vi "Read Message Box.vi"(9 "MessageBox in":refnum<class "MessageBox.lvclass">) -> (3 "MessageBox out":refnum<class "MessageBox.lvclass">, 4 "Message Box":refnum<vi>)   [LabVIEW 2014, in "Raspberry Pi Compatible Compiler for LabVIEW.lvlib" / "MessageBox.lvclass"]
uses:
  MessageBox.lvclass
  MessageBox.lvclass/MessageBox.ctl
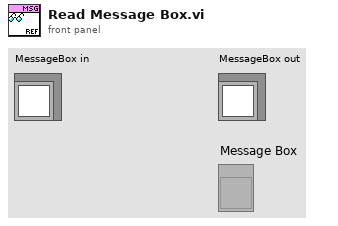
[diagram p1: front panel]
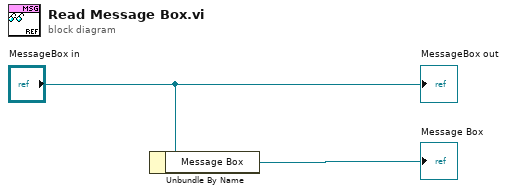
[diagram p0: block diagram]
diagram:
  n1 = Unbundle By Name("MessageBox in") -> ("Message Box"=→"Message Box":refnum<vi>)
  "MessageBox out" <- "MessageBox in"
